vi "adquirir datos audio.vi"() -> ()   [LabVIEW 2011]
panel:
  out "Waveform Graph":waveform(dbl)[](graph)
  in  "Path":path
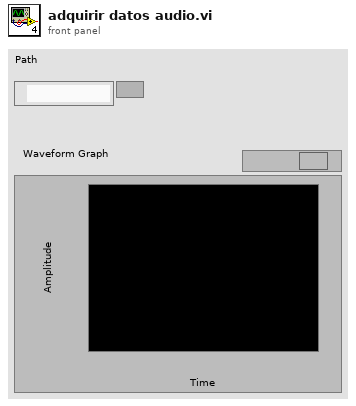
[diagram p1: front panel]
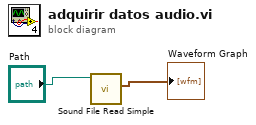
[diagram p0: block diagram]
diagram:
  n1 = call <vilib>:"Sound File Read Simple.vi"("path"="Path") -> ("data"=→"Waveform Graph":waveform(dbl)[])  [unwired: 7 in, 3 out]
